vi "RC_Client Client 2.vi"(8 "error in (no error)":errorcluster, 11 "RC Type":T1) -> (0 "error out":errorcluster)   [LabVIEW 2019, in "RemoteControl.lvclass"]
uses:
  RemoteControl.lvclass
  Typedefs/RC Com Type--enum.ctl
  1512112c-1ac8-4087-968b-87ccc04a0a5c.vi
  1512112c-1ac8-4087-968b-87ccc04a0a5c.vi/f9e71f77-168e-4138-93a7-c1df0d7b0d33.vi
  <vilib>/Utility/LVClass/Get LV Class Name.vi
  <vilib>/JDP Science/JSONtext/JSON text to Variant.vi
  <vilib>/JDP Science/JSONtext/LVClass Serializer/JSONtext LVClass Serializer.lvclass
panel:
  in  "milliseconds to wait":u32
  out "time (1 message) (ms)":u32
  out "messsages/s":dbl
  in  "remote port":u16=6341
  in  "address":string
  out "Parse Response":string
  out "Messages":i32
  in  "Stop":bool
  out "Command reponse":string
  out "Command":string
  out "commands":string[](array[string])
  # "CLIENT (API)"
  # "Connection info"
  # "Message Sent"
  # "Message Received"
  # "Metrics"
  # "client 2"
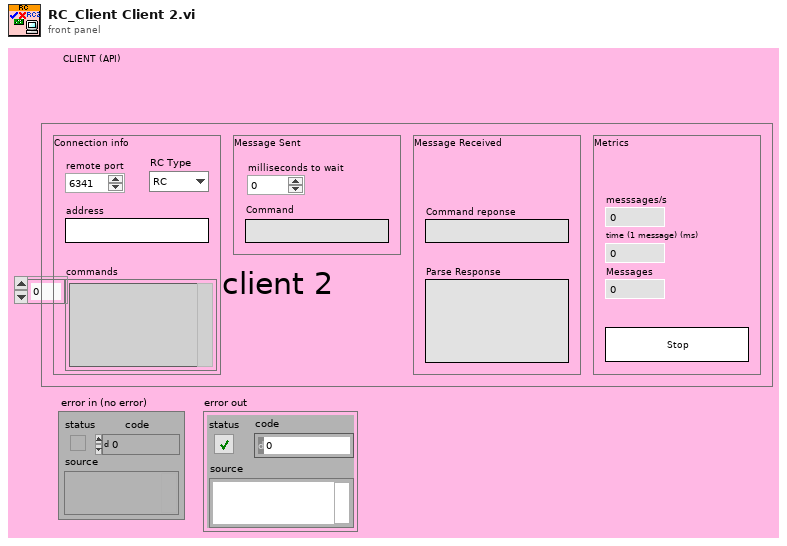
[diagram p1: front panel]
types:
  T1 = typedef "RemoteControl.lvclass/RC Com Type--enum.ctl" = enum16{"RC", "STM", "ZMQ"}
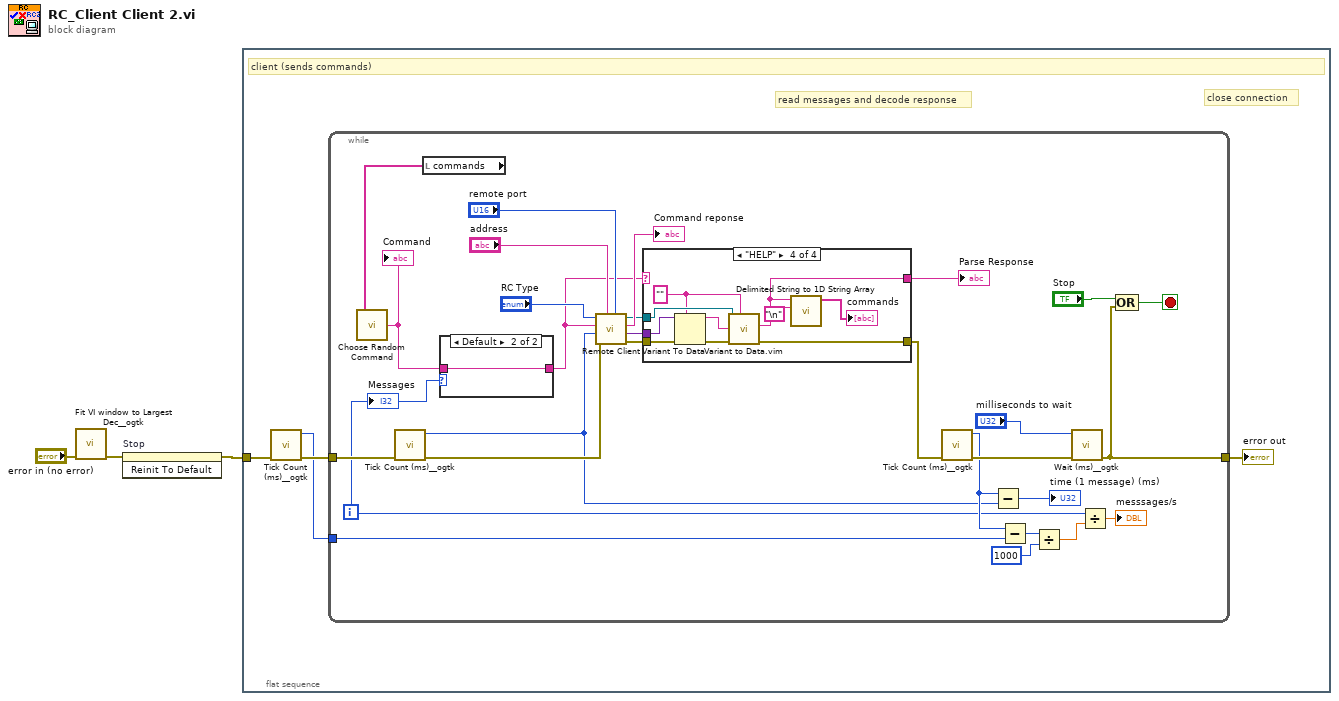
[diagram p0: block diagram]
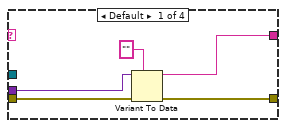
[diagram p2: hidden frame]
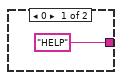
[diagram p5: hidden frame]
diagram:
  n1 = call <userlib>:"Fit VI window to Largest Dec__ogtk.vi"("error in (no error)"="error in (no error)") -> ("error out"=w3:errorcluster)  [unwired: 5 in, 1 out]
  n2 = invoke on="Stop" class="Bool" method="Reinit To Default"(error in=w3) -> (error out=w2:errorcluster)  [unwired: 2 in, 2 out]
  n3 = flat-sequence {
    tunnel: w2 -> [w4]
    frame #0 {
      # "close connection"
      # "read messages and decode response"
      # "client (sends commands)"
      n4 = call <userlib>:"Tick Count (ms)__ogtk.vi"("error in (no error)"=w4) -> ("error out"=w7:errorcluster, "millisecond timer value"=w6:u32)  [unwired: 9 in]
      n5 = while {
        tunnel: [w29] -> w5
        tunnel: w7 -> [w32]
        tunnel: w6 -> [w24]
        i -> [w21]
        stop <- w35 stop-if-true
        n6 = call <userlib>:"Tick Count (ms)__ogtk.vi"("error in (no error)"=w32) -> ("error out"=w22:errorcluster, "millisecond timer value"=w15:u32)  [unwired: 9 in]
        n7 = local read "commands"() -> (w17:string[])
        n8 = call "Choose Random Command.vi"("Array"=w17) -> ("String"=w16:string)
        "Command" <- w16
        n9 = case shown="Default" w21 {
          tunnel: ["HELP" ("Command") w56] -> w8
          tunnel: w16 -> [_ w56]
          frame 0 {
          }
          frame Default {
          }
        }
        n10 = call "Remote Client.vi"("Port"="remote port", "address"="address", "error in (no error)"=w22, "Data"=w15, "Command"=w8, "RC Type"="RC Type") -> ("error out"=w12:errorcluster, "Data out"=w13:variant, "Command out"=→"Command reponse":string, "RemoteControl out"=w11:refnum<class "RemoteControl.lvclass">)  [unwired: 2 in]
        n11 = case shown="\"HELP\"" w8 {
          selector: w8 -> [_ w41 w43 _]
          tunnel: [w36 w41 w43 w46] -> w10
          tunnel: w11 -> [_ _ _ w49]
          tunnel: w13 -> [w40 _ _ w54]
          tunnel: [w37 w42 w44 w47] -> w9
          tunnel: w12 -> [w38 w42 w44 w53]
          frame Default {
            n12 = Variant To Data(error in=w38, type="", Variant=w40) -> (data=w36:string, error out=w37:errorcluster)
          }
          frame "open" {
          }
          frame "close" {
          }
          frame "HELP" {
            w48 = ""
            n13 = Variant To Data(error in=w53, type=w48, Variant=w54) -> (data=w50:string, error out=w51:errorcluster)
            n14 = call "Variant to Data.vim"("Data Type"=w48, "error in (no error)"=w51, "Data in"=w50, "RemoteControl in"=w49) -> ("error out"=w47:errorcluster, "Data out"=w46:string)  [unwired: 5 in, 1 out]
            n15 = call <vilib>:"Delimited String to 1D String Array.vi"("delimiter"="\n", "delimited string"=w46) -> ("string array"=→"commands":string[])  [unwired: 9 in]
          }
        }
        "Parse Response" <- w10
        n16 = call <userlib>:"Tick Count (ms)__ogtk.vi"("error in (no error)"=w9) -> ("error out"=w31:errorcluster, "millisecond timer value"=w26:u32)  [unwired: 9 in]
        n17 = Subtract(x=w26, y=w15) -> (x-y=→"time (1 message) (ms)":u32)
        n18 = Subtract(x=w26, y=w24) -> (x-y=w25:u32)
        n19 = Divide(x=w25, y=u32 1000) -> (x/y=w34:dbl)
        n20 = call <userlib>:"Wait (ms)__ogtk.vi"("error in (no error)"=w31, "milliseconds to wait"="milliseconds to wait") -> ("error out"=w29:errorcluster)  [unwired: 8 in, 1 out]
        n21 = Divide(x=w21, y=w34) -> (x/y=→"messsages/s":dbl)
        n22 = Compound Arithmetic op=OR("Stop", w29) -> (w35:bool)
        "Messages" <- w21
      }
      "error out" <- w5
    }
  }
